vi "Set Console Reply(class).vi"(8 "error in (no error)":errorcluster, 10 "Console Reply.lvclass":refnum<class "Console Reply.lvclass">, 11 "EditPanel API in":refnum<class "EditPanel API.lvclass">) -> (0 "error out":errorcluster, 3 "EditPanel API out":refnum<class "EditPanel API.lvclass">)   [LabVIEW 2015, in "EditPanel API.lvlib" / "EditPanel API.lvclass"]
uses:
  EditPanel API.lvclass
  Console Reply/Console Reply/Console Reply.lvclass
  EditPanel API.lvclass/EditPanel API.ctl
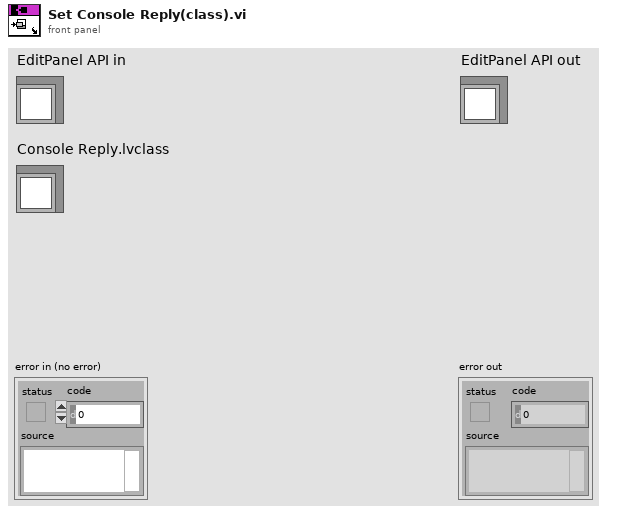
[diagram p1: front panel]
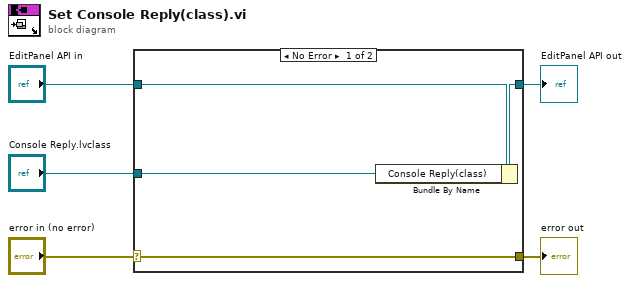
[diagram p0: block diagram]
diagram:
  n1 = case shown="No Error" "error in (no error)" {
    selector: "error in (no error)" -> [w9 w10]
    tunnel: [w9 w10] -> w4
    tunnel: [w7 w11] -> w2
    tunnel: "EditPanel API in" -> [w8 w11]
    tunnel: "Console Reply.lvclass" -> [w6 _]
    frame No Error {
      n2 = Bundle By Name(cluster=w8, "Console Reply(class)"=w6) -> (w7:refnum<class "EditPanel API.lvclass">)
    }
    frame Error {
    }
  }
  "error out" <- w4
  "EditPanel API out" <- w2
